vi "DisplacementGetSensorRawValue.vi"(10 "Sensor":u8, 11 "DisplacementSample":T1) -> (2 "Value":i32)   [LabVIEW 2018]
uses:
  DisplacementSample.ctl
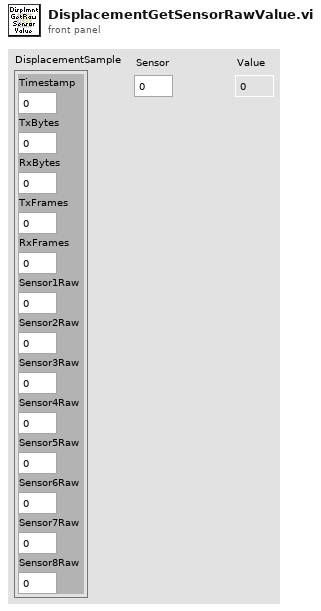
[diagram p1: front panel]
types:
  T1 = typedef "DisplacementSample.ctl" = cluster{"Timestamp":u64, "TxBytes":u64, "RxBytes":u64, "TxFrames":u64, "RxFrames":u64, "Sensor1Raw":i32, "Sensor2Raw":i32, "Sensor3Raw":i32, "Sensor4Raw":i32, "Sensor5Raw":i32, "Sensor6Raw":i32, "Sensor7Raw":i32, "Sensor8Raw":i32}
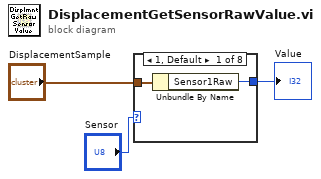
[diagram p0: block diagram]
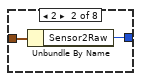
[diagram p2: hidden frame]
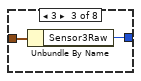
[diagram p3: hidden frame]
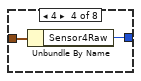
[diagram p4: hidden frame]
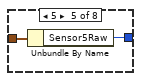
[diagram p5: hidden frame]
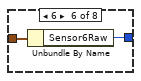
[diagram p6: hidden frame]
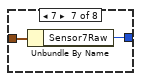
[diagram p7: hidden frame]
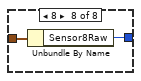
[diagram p8: hidden frame]
diagram:
  n1 = case shown="1, Default" "Sensor" {
    tunnel: "DisplacementSample" -> [w5 w7 w9 w11 w13 w15 w17 w19]
    tunnel: [w4 w6 w8 w10 w12 w14 w16 w18] -> w2
    frame 1, Default {
      n2 = Unbundle By Name(w5) -> ("Sensor1Raw"=w4:i32)
    }
    frame 2 {
      n3 = Unbundle By Name(w7) -> ("Sensor2Raw"=w6:i32)
    }
    frame 3 {
      n4 = Unbundle By Name(w9) -> ("Sensor3Raw"=w8:i32)
    }
    frame 4 {
      n5 = Unbundle By Name(w11) -> ("Sensor4Raw"=w10:i32)
    }
    frame 5 {
      n6 = Unbundle By Name(w13) -> ("Sensor5Raw"=w12:i32)
    }
    frame 6 {
      n7 = Unbundle By Name(w15) -> ("Sensor6Raw"=w14:i32)
    }
    frame 7 {
      n8 = Unbundle By Name(w17) -> ("Sensor7Raw"=w16:i32)
    }
    frame 8 {
      n9 = Unbundle By Name(w19) -> ("Sensor8Raw"=w18:i32)
    }
  }
  "Value" <- w2
